vi "Configure Power Analysis (Power Supply Rejection Ratio).vi"(7 "Vertical Scale (100)":dbl=100.0, 8 "error in (no error)":errorcluster, 9 "End Sweep Frequency (100000 Hz)":i32(ring)=100000 items=["10"=10, "100"=100, "1000"=1000, "10000"=10000, "100000"=100000, "1000000"=1000000, "10000000"=10000000, "20000000"=20000000], 10 "Start Sweep Frequency (100 Hz)":i32(ring)=100 items=["1"=1, "10"=10, "100"=100, "1000"=1000, "10000"=10000, "100000"=100000, "1000000"=1000000, "10000000"=10000000], 11 "VISA resource name":refnum<visa-resource-name>) -> (0 "error out":errorcluster, 3 "VISA resource name out":refnum<visa-resource-name>)   [LabVIEW 2017, in "Agilent 2000 3000 X-Series.lvlib"]
doc: "Configures the power supply rejection ratio (PSRR) analysis.\n\n<B>Note(s):</B>\nThis VI is not supported by EDUX1052A/G, DSOX1202A/G, DSOX1204A/G models\nThe Power Supply Rejection Ratio (PSRR) test is used to determine how well a voltage regulator rejects ripple noise over different frequency range.\n\nThis analysis provides a signal from the oscilloscope's waveform generator that sweeps its frequency. This signal is used to inject ripple to the DC voltage that feeds the voltage regulator.\n\nThe AC RMS ratio of the input over the output is measured and is plotted over the range of frequencies."
uses:
  Agilent 2000 3000 X-Series.lvlib
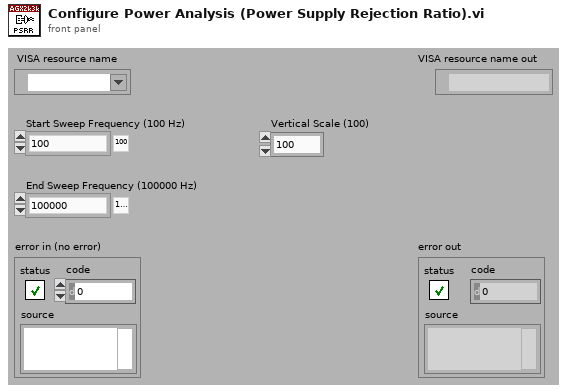
[diagram p1: front panel]
types:
  T1 = typedef "Agilent 2000 3000 X-Series.lvlib/Extended User Data.ctl" = cluster{"X-Series Mode":u16, "Acquisition Type (0: Normal)":i32}
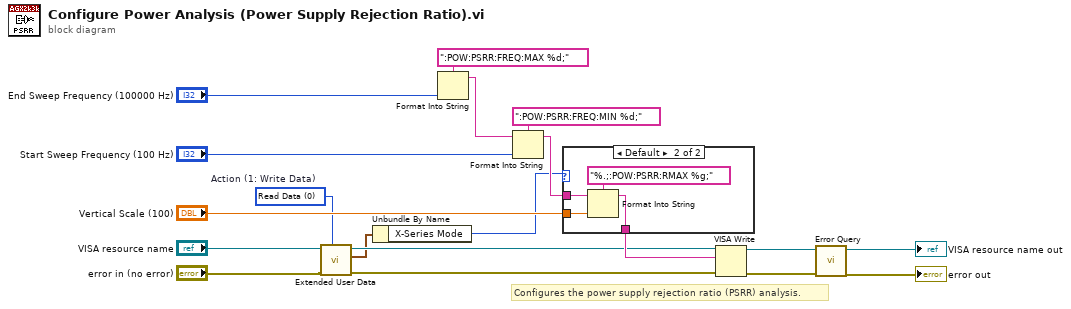
[diagram p0: block diagram]
diagram:
  w3 = 0 items=["Read Data", "Write Data", "Clear Data", "Clear ALL Data"]  # Action (1: Write Data)
  # "Configures the power supply rejection ratio (PSRR) analysis."
  n1 = call "Extended User Data.vi"("Action (1: Write Data)"=w3, "error in (no error)"="error in (no error)", "VISA resource name in"="VISA resource name") -> ("error out"=w4:errorcluster, "User Data Out"=w2:T1, "VISA resource name out"=w5:refnum<visa-resource-name>)  [unwired: 6 in]
  n2 = Unbundle By Name(w2) -> ("X-Series Mode"=w1:u16)
  n3 = Format Into String(format string=":POW:PSRR:FREQ:MAX %d;", "End Sweep Frequency (100000 Hz)") -> (resulting string=w17:string)  [unwired: 2 in, 1 out]
  n4 = Format Into String(format string=":POW:PSRR:FREQ:MIN %d;", initial string=w17, "Start Sweep Frequency (100 Hz)") -> (resulting string=w14:string)  [unwired: 1 in, 1 out]
  n5 = case shown="Default" w1 {
    tunnel: w14 -> [w20 w24]
    tunnel: "Vertical Scale (100)" -> [_ w22]
    tunnel: [w20 w21] -> w8
    frame 82..101 {
    }
    frame Default {
      n6 = Format Into String(format string="%.;:POW:PSRR:RMAX %g;", initial string=w24, w22) -> (resulting string=w21:string)  [unwired: 1 in, 1 out]
    }
  }
  n7 = VISA Write(VISA resource name=w5, write buffer=w8, error in (no error)=w4) -> (VISA resource name out=w12:refnum<visa-resource-name>, error out=w11:errorcluster)  [unwired: 1 out]
  n8 = call "Error Query.vi"("error in (no error)"=w11, "VISA resource name"=w12) -> ("error out"=→"error out":errorcluster, "VISA resource name out"=→"VISA resource name out":refnum<visa-resource-name>)  [unwired: 8 out]
